vi "Change Camera Settings.vi"() -> ()   [LabVIEW 2013]
panel:
  out "Min SS":errorcluster
  out "Max SS":errorcluster
  out "Min Gain":errorcluster
  out "Max Gain":errorcluster
  in  "Min Gain":bool
  in  "Max Gain":bool
  in  "Min Shutter Speed":bool
  in  "Max Shutter Speed":bool
  in  "Max Shutter Speed":i32=50 min=0
  in  "Min Shutter Speed":i32=50 min=0
  in  "Max Gain":i32=50 min=0
  in  "Min Gain":i32=50 min=0
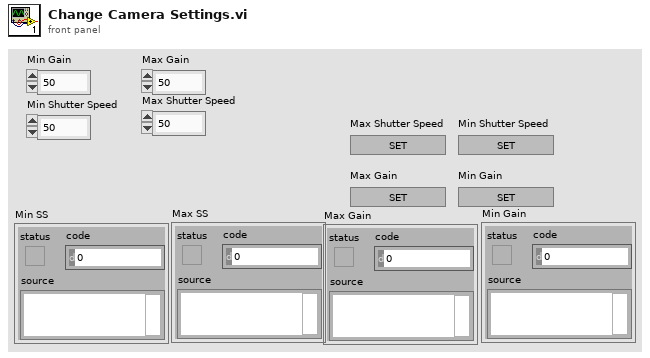
[diagram p1: front panel]
types:
  T1 = typedef "WPI_CameraDevRef.ctl" = cluster{"Camera Address":string, "CameraStatus":errorcluster, "Acquire Image Notifier":refnum<notifier>}
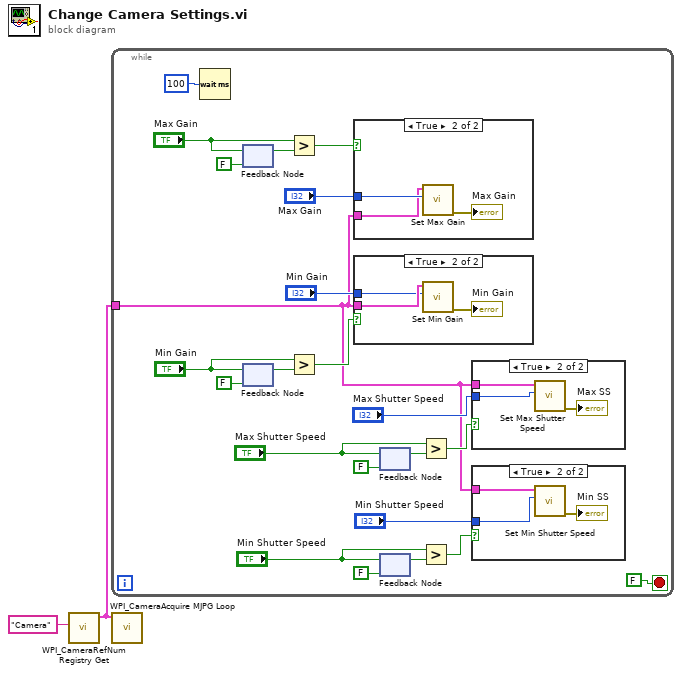
[diagram p0: block diagram]
diagram:
  n1 = call <vilib>:"WPI_CameraRefNum Registry Get.vi"("refnum name"="Camera") -> ("CameraDevRef"=w2:T1)  [unwired: 9 in, 1 out]
  n2 = while {
    tunnel: w2 -> [w3]
    stop <- FALSE stop-if-true
    n3 = Wait (ms)(milliseconds to wait=u32 100) -> ()  [unwired: 1 out]
    n4 = feedback #1(FALSE ("Max Shutter Speed")) -> (w18:bool)
    n5 = feedback-in #1("Max Gain") -> ()
    n6 = feedback #2(FALSE ("Max Shutter Speed")) -> (w13:bool)
    n7 = feedback-in #2("Min Gain") -> ()
    n8 = Greater?(x="Max Gain", y=w18) -> (0:w4:bool)
    n9 = Greater?(x="Min Gain", y=w13) -> (0:w8:bool)
    n10 = case shown="True" w4 {
      tunnel: "Max Gain" -> [_ w28]
      tunnel: w3 -> [_ w27]
      frame False {
      }
      frame True {
        n11 = call "Set Max Gain.vi"("Gain"=w28, "CameraDevRef"=w27) -> ("error out"=→"Max Gain":errorcluster)  [unwired: 8 in, 1 out]
      }
    }
    n12 = case shown="True" w8 {
      tunnel: w3 -> [_ w34]
      tunnel: "Min Gain" -> [_ w33]
      frame False {
      }
      frame True {
        n13 = call "Set Min Gain.vi"("Gain"=w33, "CameraDevRef"=w34) -> ("error out"=→"Min Gain":errorcluster)  [unwired: 8 in, 1 out]
      }
    }
    n14 = feedback-in #3("Max Shutter Speed") -> ()
    n15 = feedback #3(FALSE ("Max Shutter Speed")) -> (w21:bool)
    n16 = feedback #4(FALSE ("Max Shutter Speed")) -> (w16:bool)
    n17 = feedback-in #4("Min Shutter Speed") -> ()
    n18 = Greater?(x="Max Shutter Speed", y=w21) -> (0:w10:bool)
    n19 = Greater?(x="Min Shutter Speed", y=w16) -> (0:w7:bool)
    n20 = case shown="True" w10 {
      tunnel: "Max Shutter Speed" -> [_ w37]
      tunnel: w3 -> [_ w36]
      frame False {
      }
      frame True {
        n21 = call "Set Max Shutter Speed.vi"("Shutter Speed"=w37, "CameraDevRef"=w36) -> ("error out"=→"Max SS":errorcluster)  [unwired: 8 in, 1 out]
      }
    }
    n22 = case shown="True" w7 {
      tunnel: "Min Shutter Speed" -> [_ w31]
      tunnel: w3 -> [_ w30]
      frame False {
      }
      frame True {
        n23 = call "Set Min Shutter Speed.vi"("Shutter Speed"=w31, "CameraDevRef"=w30) -> ("error out"=→"Min SS":errorcluster)  [unwired: 8 in, 1 out]
      }
    }
  }
  n24 = call <vilib>:"WPI_CameraAcquire MJPG Loop.vi"("CameraDevRef"=w2) -> ()  [unwired: 11 in]
